vi "LAS-CTS_SingleSpotMonitorImproved.vi"() -> ()   [LabVIEW 2024]
uses:
  <vilib>/httpClient/LabVIEWHTTPClient.lvlib
panel:
  out "loop iter":i32
  out "laser iter":i32
  out "record iter":i32
  out "last file name":string
  in  "base filename":string
  in  "file number":i32 format="%03d"
  out "Waveform Chart":dbl(graph)
  in  "Post-read delay (ms)":u32
  in  "Z position (mirror mm)":string
  in  "X position (mirror mm)":string
  in  "Target ID":string
  in  "data filepath":path
  in  "Number of Pulses":i32
  out "Laser On/Off":bool
  out "Pulses Remaining":i32
  in  "# data points":i32
  in  "Keithly":refnum<visa-resource-name>
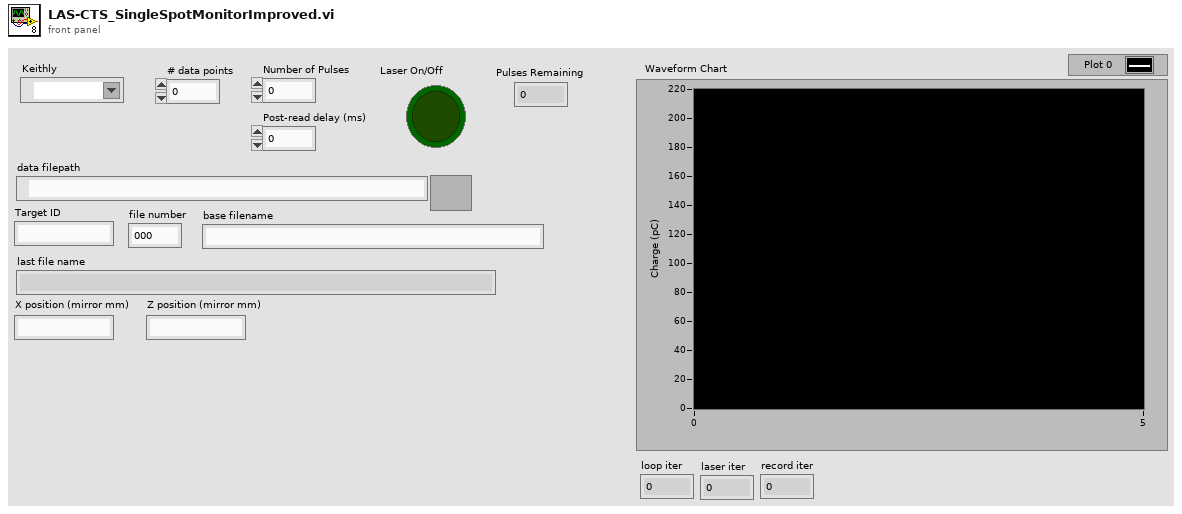
[diagram p1: front panel]
types:
  T1 = enum16{"open", "replace", "create", "open or create", "replace or create", "replace or create with confirmation"}
  T2 = typedef "LabVIEWHTTPClient.lvlib/ClientHandle.ctl" = refnum<k1>
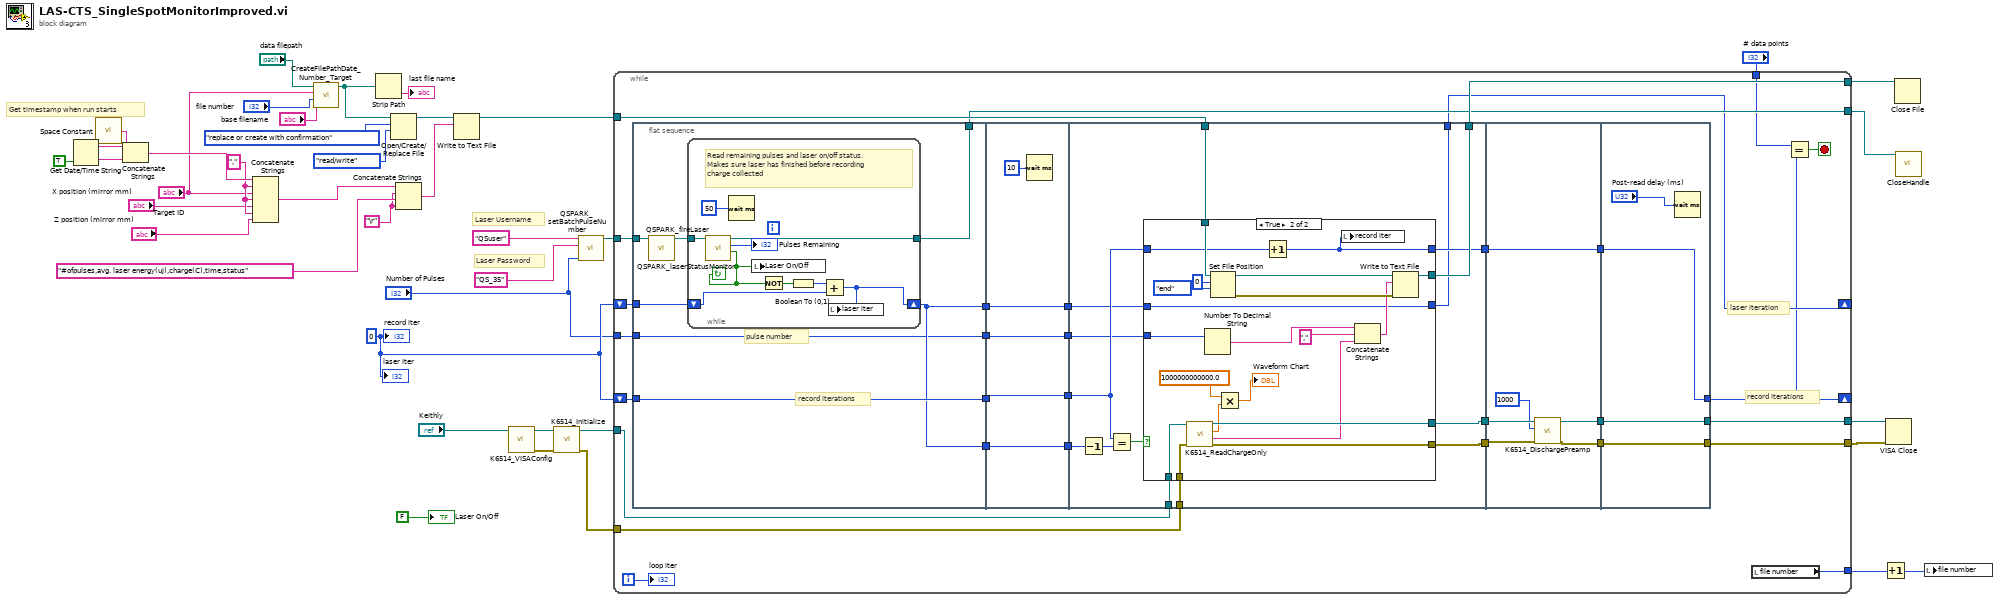
[diagram p0: block diagram]
diagram:
  w3 = 0 ("iter")
  w15 = "," ("string")
  w27 = "\r"
  # "Get timestamp when run starts"
  # "Laser Password"
  # "Laser Username"
  n1 = Get Date/Time String(want seconds? (F)=TRUE) -> (date string=w26:string, time string=w25:string)  [unwired: 2 in]
  n2 = call <vilib>:"Space Constant.vi"() -> ("String"=w24:string)
  n3 = Concatenate Strings(w26, w24, w25) -> (w22:string)
  n4 = Concatenate Strings(w22, w15, "Target ID", w15, "X position (mirror mm)", w15, "Z position (mirror mm)") -> (w21:string)
  n5 = call "CreateFilePathDate_Number_Target.vi"("base filename"="base filename", "file number"="file number", "Target ID"="Target ID", "data filepath"="data filepath") -> ("appended path"=w6:path)  [unwired: 7 in]
  n6 = Strip Path(path=w6) -> (name=→"last file name":string)  [unwired: 1 out]
  n7 = Open/Create/Replace File(file path (use dialog)=w6, operation (0:open)=T1."replace or create with confirmation", access (0:read/write)=enum16{"read/write", "read-only", "write-only"}."read/write") -> (refnum out=w30:refnum<file>)  [unwired: 3 in, 2 out]
  n8 = Concatenate Strings(w21, w27, "#ofpulses,avg. laser energy(uJ),charge(C),time,status", w27) -> (w28:string)
  n9 = Write to Text File(file (use dialog)=w30, text=w28) -> (refnum out=w20:refnum<file>)  [unwired: 2 in, 2 out]
  n10 = call "K6514_VISAConfig.vi"("VISA resource name"="Keithly") -> ("error out"=w40:errorcluster, "reference out"=w39:refnum<visa-resource-name>)  [unwired: 9 in]
  n11 = call "K6514_Initialize.vi"("error in (no error)"=w40, "VISA resource name"=w39) -> ("error out"=w33:errorcluster, "VISA resource name out"=w4:refnum<visa-resource-name>)  [unwired: 8 in]
  n12 = call "QSPARK_setBatchPulseNumber.vi"("Number of Pulses"="Number of Pulses", "password"="QS_35", "username"="QSuser") -> ("client handle out"=w35:T2)  [unwired: 8 in]
  n13 = while {
    tunnel: w35 -> [w71]
    tunnel: w33 -> [w70]
    tunnel: w20 -> [w67]
    tunnel: [w66] -> w19
    tunnel: [w65] -> w18
    tunnel: [w64] -> w17
    tunnel: [w63] -> w16
    tunnel: [w60] -> w7
    tunnel: w4 -> [w59]
    shift-right: [w50] -> _
    shift-left: w3 -> [w58]
    shift-right: [w46] -> _
    shift-left: w3 -> [w54]
    tunnel: "# data points" -> [w41]
    tunnel: "Number of Pulses" -> [w45]
    i -> [w42]
    stop <- w47 stop-if-true
    # "laser iteration"
    # "record iterations"
    n14 = flat-sequence {
      tunnel: w71 -> [w77]
      tunnel: [w76] -> w63
      tunnel: w58 -> [w75]
      tunnel: [w73] -> w56
      tunnel: [w74] -> w55
      tunnel: w54 -> [w74]
      tunnel: [w73] -> w48
      tunnel: w45 -> [w72]
      tunnel: [w72] -> w44
      tunnel: [w91] -> w57
      tunnel: w56 -> [w91]
      tunnel: w55 -> [w90]
      tunnel: [w90] -> w53
      tunnel: [w89] -> w49
      tunnel: w48 -> [w89]
      tunnel: w44 -> [w88]
      tunnel: [w88] -> w43
      tunnel: w70 -> [w106]
      tunnel: [w105] -> w69
      tunnel: [w104] -> w68
      tunnel: w67 -> [w103]
      tunnel: [w102] -> w64
      tunnel: w59 -> [w101]
      tunnel: w57 -> [w93]
      tunnel: w53 -> [w99]
      tunnel: [w98] -> w51
      tunnel: [w97] -> w50
      tunnel: w49 -> [w96]
      tunnel: w43 -> [w95]
      tunnel: w69 -> [w138]
      tunnel: w68 -> [w137]
      tunnel: [w135] -> w62
      tunnel: [w134] -> w61
      tunnel: [w133] -> w52
      tunnel: w51 -> [w133]
      tunnel: [w141] -> w65
      tunnel: [w142] -> w66
      tunnel: w62 -> [w142]
      tunnel: w61 -> [w141]
      tunnel: [w139] -> w46
      tunnel: w52 -> [w139]
      frame #0 {
        # "pulse number"
        # "record iterations"
        n15 = call "QSPARK_fireLaser.vi"("client handle"=w77) -> ("client handle out"=w78:T2)  [unwired: 10 in]
        n16 = while {
          tunnel: w78 -> [w86]
          tunnel: [w85] -> w76
          shift-right: [w79] -> w73
          shift-left: w75 -> [w80]
          stop <- w83 continue-if-true
          # "Read remaining pulses and laser on/off status. \nMakes sure laser has finished before recording \ncharge collected"
          n17 = call "QSPARK_laserStatusMonitor.vi"("client handle"=w86) -> ("laser on?"=w83:bool, "remaining pulses"=→"Pulses Remaining":i32, "client handle out"=w85:T2)  [unwired: 8 in]
          n18 = Wait (ms)(milliseconds to wait=u32 50 ("millisecond multiple")) -> ()  [unwired: 1 out]
          n19 = local write "Laser On/Off"(w83) -> ()
          n20 = Not(x=w83) -> (.not. x?=w82:bool)
          n21 = Boolean To (0,1)(Boolean=w82) -> (0, 1=w81:i16)
          n22 = Add(x=w81, y=w80) -> (x+y=w79:i32)
          n23 = local write "laser iter"(w79) -> ()
        }
      }
      frame #1 {
        n24 = Wait (ms)(milliseconds to wait=u32 10) -> ()  [unwired: 1 out]
      }
      frame #2 {
        n25 = Decrement(x=w93) -> (x-1=w94:i32)
        n26 = Equal?(x=w99, y=w94) -> (x = y?=w100:bool)
        n27 = case shown="True" w100 {
          tunnel: w106 -> [w108 w125]
          tunnel: [w108 w124] -> w105
          tunnel: [w107 w123] -> w104
          tunnel: w103 -> [w111 w122]
          tunnel: [w111 w121] -> w102
          tunnel: w101 -> [w107 w117]
          tunnel: w99 -> [w110 w116]
          tunnel: [w110 w112] -> w98
          tunnel: [w109 w115] -> w97
          tunnel: w96 -> [w109 w115]
          tunnel: w95 -> [_ w113]
          frame False {
          }
          frame True {
            n28 = call "K6514_ReadChargeOnly.vi"("error in (no error)"=w125, "VISA resource name"=w117) -> ("error out"=w124:errorcluster, "Response"=w114:string, "charge(C)"=w120:dbl, "VISA resource name out"=w123:refnum<visa-resource-name>)  [unwired: 5 in]
            n29 = Number To Decimal String(number=w113) -> (decimal integer string=w127:string)  [unwired: 1 in]
            n30 = Set File Position(offset (in bytes) (0)=i64 0, refnum=w122, from (0:start)=enum16{"start", "end", "current"}."end") -> (refnum out=w129:refnum<file>, error out=w132:errorcluster)  [unwired: 1 in]
            n31 = Multiply(x=1000000000000.0, y=w120) -> (x*y=→"Waveform Chart":dbl)
            n32 = Increment(x=w116) -> (x+1=w112:i32)
            n33 = local write "record iter"(w112) -> ()
            n34 = Concatenate Strings(w127, "," ("string"), w114) -> (w128:string)
            n35 = Write to Text File(file (use dialog)=w129, text=w128, error in=w132) -> (refnum out=w121:refnum<file>)  [unwired: 1 in, 2 out]
          }
        }
      }
      frame #3 {
        n36 = call "K6514_DischargePreamp.vi"("error in (no error)"=w138, "discharge time (ms)"=1000, "VISA resource name in"=w137) -> ("error out"=w134:errorcluster, "VISA resource name out"=w135:refnum<visa-resource-name>)  [unwired: 7 in]
      }
      frame #4 {
        n37 = Wait (ms)(milliseconds to wait="Post-read delay (ms)") -> ()  [unwired: 1 out]
      }
    }
    n38 = local read "file number"() -> (w60:i32)
    n39 = Equal?(x=w41, y=w46) -> (x = y?=w47:bool)
    "loop iter" <- w42
  }
  n40 = Increment(x=w7) -> (x+1=w8:i32)
  n41 = VISA Close(VISA resource name=w19, error in (no error)=w18) -> ()  [unwired: 1 out]
  n42 = Close File(refnum=w17) -> ()  [unwired: 1 in, 2 out]
  n43 = call <vilib>:"CloseHandle.vi"("client handle"=w16) -> ()  [unwired: 14 in, 1 out]
  n44 = local write "file number"(w8) -> ()
  "Laser On/Off" <- FALSE ("Laser On/Off")
  "record iter" <- w3
  "laser iter" <- w3
